vi "ep_File Descr Inf to String.vi"(8 "error in":errorcluster, 10 "initial string":string, 11 "task in":T1={"file refnums"=[], "Data Object"=refnum, "config info"={"station_name"="", "rec_dev_id"="", "rev_year"=1999.0, "TT"=0, "##A"=0, "##D"=0, "analog channel info"=[], "status channel info"=[], "lf"=-inf, "nrates"=65535, "samp info"=[], "initial timestamp"=timestamp(0 s since 1904-01-01), "trigger timestamp"=timestamp(0 s since 1904-01-01), "ft"=enum."Binary", "timemult"=1.0}, "public inf content"={"Source"="", "Record Type"=enum."Fault", "Phase ID"="", "Event Description"="", "Device ID"="", "Distance of Fault"=-1.0, "Distance Unit"=enum."Miles", "Max_Current"=inf, "Min_Current"=-inf, "Max_Voltage"=inf, "Min_Voltage"=-inf, "EventNoteCount"=0, "Event Information"=[]}, "private inf content"=[], "internal buffers"={"start index"=1, "config to public inf"=enum."disabled", "static config info"="", "static file_des record inf"="", "static file_des channel inf"="", "public inf"="", "private inf"=""}} {"public inf content"."Event Information"."min sample number" max=9999999999; "public inf content"."Event Information"."max sample number" max=9999999999; "config info"."nrates" max=999; "config info"."status channel info"."Dn" min=1 max=999999; "config info"."analog channel info"."An" min=1 max=999999; "config info"."trigger timestamp" format="%<%H:%M:%S%6u\n%d/%m/%Y>T"; "config info"."initial timestamp" format="%<%H:%M:%S%6u\n%d/%m/%Y>T"; "config info"."##D" max=999999; "config info"."##A" max=999999; "config info"."TT" min=1 max=999999; "config info"."rev_year" min=1999.0 max=1999.0}) -> (0 "error out":errorcluster, 2 "file_des inf appended":string, 3 "task out":T1={"file refnums"=[], "Data Object"=refnum, "config info"={"station_name"="", "rec_dev_id"="", "rev_year"=1999.0, "TT"=0, "##A"=0, "##D"=0, "analog channel info"=[], "status channel info"=[], "lf"=-inf, "nrates"=65535, "samp info"=[], "initial timestamp"=timestamp(0 s since 1904-01-01), "trigger timestamp"=timestamp(0 s since 1904-01-01), "ft"=enum."Binary", "timemult"=1.0}, "public inf content"={"Source"="", "Record Type"=enum."Fault", "Phase ID"="", "Event Description"="", "Device ID"="", "Distance of Fault"=-1.0, "Distance Unit"=enum."Miles", "Max_Current"=inf, "Min_Current"=-inf, "Max_Voltage"=inf, "Min_Voltage"=-inf, "EventNoteCount"=0, "Event Information"=[]}, "private inf content"=[], "internal buffers"={"start index"=1, "config to public inf"=enum."disabled", "static config info"="", "static file_des record inf"="", "static file_des channel inf"="", "public inf"="", "private inf"=""}} {"public inf content"."Event Information"."min sample number" max=9999999999; "public inf content"."Event Information"."max sample number" max=9999999999; "config info"."nrates" max=999; "config info"."status channel info"."Dn" min=1 max=999999; "config info"."analog channel info"."An" min=1 max=999999; "config info"."trigger timestamp" format="%<%H:%M:%S%6u\n%d/%m/%Y>T"; "config info"."initial timestamp" format="%<%H:%M:%S%6u\n%d/%m/%Y>T"; "config info"."##D" max=999999; "config info"."##A" max=999999; "config info"."TT" min=1 max=999999; "config info"."rev_year" min=1999.0 max=1999.0})   [LabVIEW 2014, in "NI_EP_COMTRADE.lvlib"]
uses:
  <vilib>/addons/Electrical Power/File IO/NI_EP_COMTRADE.lvlib
  <vilib>/addons/Electrical Power/File IO/COMTRADE/typedefs/ep_Task.ctl
  <vilib>/addons/Electrical Power/File IO/COMTRADE/typedefs/ep_Config Info.ctl
  <vilib>/addons/Electrical Power/File IO/COMTRADE/typedefs/ep_Analog Channel Info.ctl
  <vilib>/addons/Electrical Power/File IO/COMTRADE/typedefs/ep_Status Channel Info.ctl
  <vilib>/addons/Electrical Power/File IO/COMTRADE/typedefs/ep_File Format.ctl
  <vilib>/addons/Electrical Power/File IO/COMTRADE/typedefs/ep_Public Inf Content.ctl
  <vilib>/addons/Electrical Power/File IO/COMTRADE/typedefs/ep_Public Event Inf.ctl
  <vilib>/addons/Electrical Power/File IO/COMTRADE/typedefs/ep_Private Inf Content.ctl
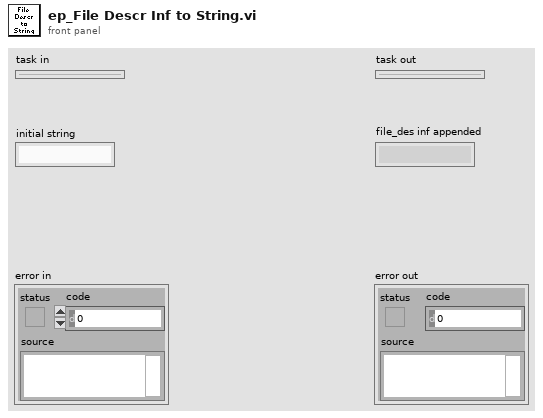
[diagram p1: front panel]
types:
  T1 = typedef "NI_EP_COMTRADE.lvlib/ep_Task.ctl" = cluster{"file refnums":refnum<file>[], "Data Object":refnum<k20>, "config info":T2, "public inf content":T6, "private inf content":T8, "internal buffers":cluster{"start index":u32, "config to public inf":enum16{"disabled", "enabled", "buffered"}, "static config info":string, "static file_des record inf":string, "static file_des channel inf":string, "public inf":string, "private inf":string}}
  T2 = typedef "NI_EP_COMTRADE.lvlib/ep_Config Info.ctl" = cluster{"station_name":string, "rec_dev_id":string, "rev_year":dbl, "TT":u32, "##A":u32, "##D":u32, "analog channel info":T3[], "status channel info":T4[], "lf":sgl, "nrates":u16, "samp info":cluster{"samp":sgl, "endsamp":u32}[], "initial timestamp":timestamp, "trigger timestamp":timestamp, "ft":T5, "timemult":sgl}
  T3 = typedef "NI_EP_COMTRADE.lvlib/ep_Analog Channel Info.ctl" = cluster{"An":u32, "ch_id":string, "ph":string, "ccbm":string, "uu":string, "a":sgl, "b":sgl, "skew":sgl, "min":i32, "max":i32, "primary":sgl, "secondary":sgl, "PS":enum16{"P", "S"}}
  T4 = typedef "NI_EP_COMTRADE.lvlib/ep_Status Channel Info.ctl" = cluster{"Dn":u32, "ch_id":string, "ph":string, "ccbm":string, "Y":bool}
  T5 = typedef "NI_EP_COMTRADE.lvlib/ep_File Format.ctl" = enum16{"ASCII", "Binary"}
  T6 = typedef "NI_EP_COMTRADE.lvlib/ep_Public Inf Content.ctl" = cluster{"Source":string, "Record Type":enum16{"Fault", "Unknown", "Misoperation", "Close", "Trip", "Reclose", "Power swing", "Simulation"}, "Phase ID":string, "Event Description":string, "Device ID":string, "Distance of Fault":dbl, "Distance Unit":enum16{"Miles", "Kilometers", "Percent of line", "Percent of setting", "Ohms"}, "Max_Current":dbl, "Min_Current":dbl, "Max_Voltage":dbl, "Min_Voltage":dbl, "EventNoteCount":u32, "Event Information":T7[]}
  T7 = typedef "NI_EP_COMTRADE.lvlib/ep_Public Event Inf.ctl" = cluster{"channel number":u32, "max value":dbl, "min value":dbl, "max sample number":u64, "min sample number":u64, "max sample text":string[], "min sample text":string[]}
  T8 = typedef "NI_EP_COMTRADE.lvlib/ep_Private Inf Content.ctl" = cluster{"Section Header":string, "Entry Names":string[], "Entry Values":string[]}[]
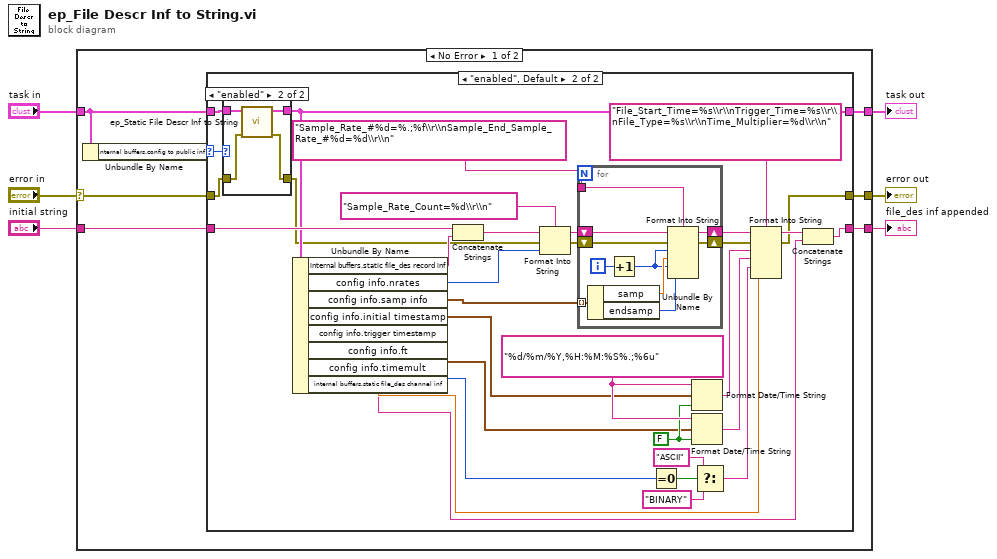
[diagram p0: block diagram]
diagram:
  n1 = case shown="No Error" "error in" {
    selector: "error in" -> [w8 w68]
    tunnel: [w9 w68] -> w5
    tunnel: "task in" -> [w13 w67]
    tunnel: [w11 w67] -> w3
    tunnel: "initial string" -> [w12 w66]
    tunnel: [w10 w66] -> w1
    frame No Error {
      n2 = Unbundle By Name(w13) -> ("internal buffers.config to public inf"=w7:enum16{"disabled", "enabled", "buffered"})
      n3 = case shown="\"enabled\", Default" w7 {
        selector: w7 -> [_ w20]
        tunnel: w13 -> [w16 w49]
        tunnel: w12 -> [w14 w48]
        tunnel: [w16 w23] -> w11
        tunnel: [w14 w22] -> w10
        tunnel: [w15 w21] -> w9
        tunnel: w8 -> [w15 w19]
        frame "disabled" {
        }
        frame "enabled", Default {
          w33 = FALSE ("UTC format")
          w45 = "%d/%m/%Y,%H:%M:%S%.;%6u" ("time format string (%c)")
          n4 = case shown="\"enabled\"" w20 {
            tunnel: w49 -> [w61 w65]
            tunnel: [w61 w64] -> w23
            tunnel: w19 -> [w60 w63]
            tunnel: [w60 w62] -> w18
            frame "buffered", Default {
            }
            frame "enabled" {
              n5 = call <vilib>:"ep_Static File Descr Inf to String.vi"("error in"=w63, "task in"=w65) -> ("error out"=w62:errorcluster, "task out"=w64:T1)  [unwired: 8 in]
            }
          }
          n6 = Unbundle By Name(w23) -> ("internal buffers.static file_des record inf"=w47:string, "config info.nrates"=w32:u16, "config info.samp info"=w30:cluster{"samp":sgl, "endsamp":u32}[], "config info.initial timestamp"=w28:timestamp, "config info.trigger timestamp"=w27:timestamp, "config info.ft"=w29:T5, "config info.timemult"=w26:sgl, "internal buffers.static file_des channel inf"=w24:string)
          n7 = Concatenate Strings(w48, w47) -> (w31:string)
          n8 = Format Into String(format string="Sample_Rate_Count=%d\\r\\n", initial string=w31, error in=w18, w32) -> (resulting string=w36:string, error out=w34:errorcluster)
          n9 = for {
            shift-right: [w57] -> w37
            shift-left: w36 -> [w59]
            shift-right: [w56] -> w35
            shift-left: w34 -> [w58]
            tunnel: w30 -> [w51] mode=indexing
            tunnel: "Sample_Rate_#%d=%.;%f\\r\\nSample_End_Sample_Rate_#%d=%d\\r\\n" ("format string") -> [w50]
            i -> [w54]
            n10 = Unbundle By Name(w51) -> ("samp"=w55:sgl, "endsamp"=w53:u32)
            n11 = Increment(x=w54) -> (x+1=w52:i32)
            n12 = Format Into String(format string=w50, initial string=w59, error in=w58, w52, w55, w52, w53) -> (resulting string=w57:string, error out=w56:errorcluster)
          }
          n13 = Equal To 0?(x=w29) -> (x = 0?=w42:bool)
          n14 = Format Date/Time String(time format string (%c)=w45, seconds (now)=w28, UTC format=w33) -> (date/time string=w44:string)
          n15 = Format Date/Time String(time format string (%c)=w45, seconds (now)=w27, UTC format=w33) -> (date/time string=w43:string)
          n16 = Select(t="ASCII", s=w42, f="BINARY") -> (s? t:f=w39:string)
          n17 = Format Into String(format string="File_Start_Time=%s\\r\\nTrigger_Time=%s\\r\\nFile_Type=%s\\r\\nTime_Multiplier=%d\\r\\n", initial string=w37, error in=w35, w44, w43, w39, w26) -> (resulting string=w25:string, error out=w21:errorcluster)
          n18 = Concatenate Strings(w25, w24) -> (w22:string)
        }
      }
    }
    frame Error {
    }
  }
  "file_des inf appended" <- w1
  "task out" <- w3
  "error out" <- w5
